vi "AR Drone + Simple nav.vi"() -> ()   [LabVIEW 2014]
doc: "Very simple example showing how to use the base VIs to control the AR Drone and receive and display video data."
uses:
  Others/Control cluster.ctl
  <vilib>/LVH/AR Drone Toolkit/Decode NavData/Typedefs/NavData Demo.ctl
  Global.vi
  <vilib>/LVH/AR Drone Toolkit/AR Drone.lvlib
panel:
  in  "milliseconds to wait":u32=5
  out "Delay (ms)":u32
  in  "Takeoff/Land":bool
  out "Video Stream 2":picture
  in  "Setup Parameters":T1={"Drone IP address"="192.168.1.1", "Home IP address"="192.168.1.2", "Flight Mode"=enum."INDOOR MODE", "Mounted Hull"=enum."INDOOR HULL", "Video Camera"=0, "Max Altitude (m)"=3.0, "Max Pitch and Roll Angle (deg)"=10.0, "Max Vertical Speed (m/s)"=0.7, "Max Yaw Speed (deg/s)"=100.0} {"Video Camera" items=["Bottom Camera"=1, "Front Camera"=0, "Front in Bottom"=3, "Bottom in Front"=2]}
  in  "stop":bool
  out "Loop error":errorcluster
  out "Loop count":i32
  out "Battery Remaining 2":dbl(slide) scale=0.0..100.0
  out "NavData Out 2":T2
  out "Control Cluster":T3 {"Yaw Speed" scale=-1.0..1.0; "Vertical Speed" scale=-1.0..1.0; "Pitch" scale=-1.0..1.0; "Roll" scale=-1.0..1.0}
  in  "Emergency Landing":bool
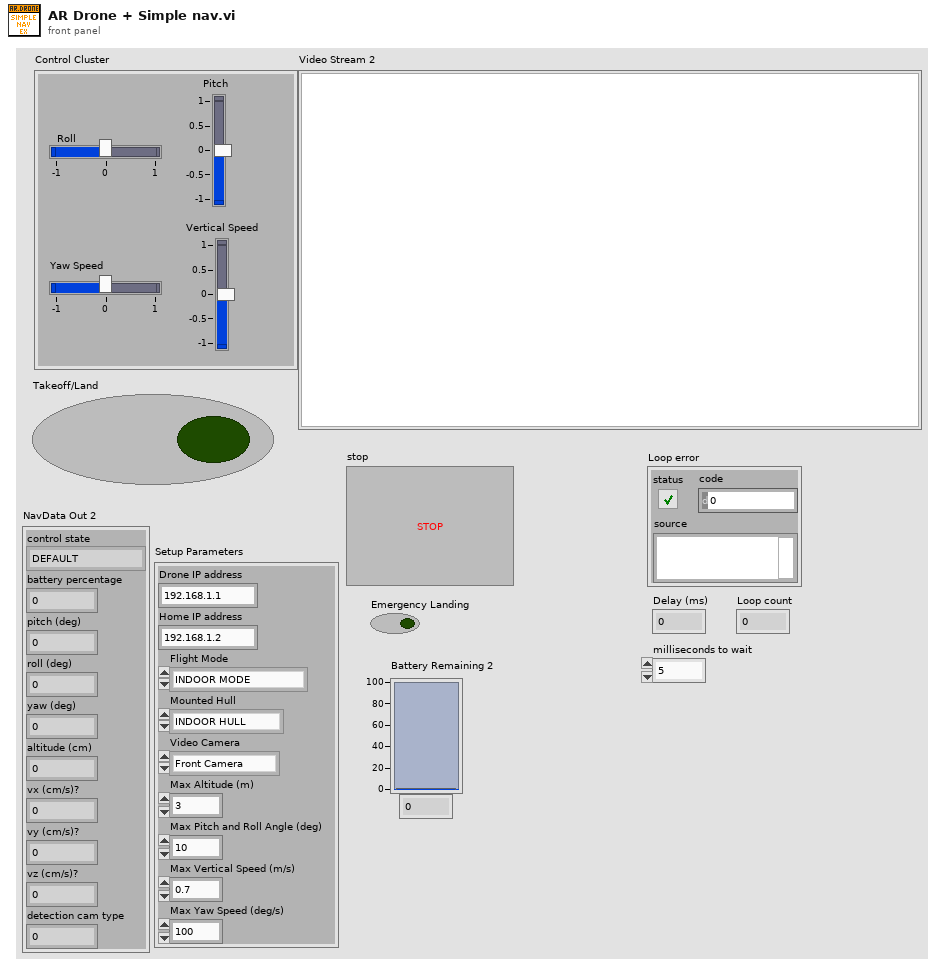
[diagram p1: front panel]
types:
  T1 = cluster{"Drone IP address":string, "Home IP address":string, "Flight Mode":enum8{"OUTDOOR MODE", "INDOOR MODE"}, "Mounted Hull":enum8{"OUTDOOR HULL", "INDOOR HULL"}, "Video Camera":u8, "Max Altitude (m)":sgl, "Max Pitch and Roll Angle (deg)":sgl, "Max Vertical Speed (m/s)":sgl, "Max Yaw Speed (deg/s)":sgl}
  T2 = typedef "AR Drone.lvlib/NavData Demo.ctl" = cluster{"control state":enum32{"DEFAULT", "INIT", "LANDING", "FLYING", "HOVERING", "TEST", "TRANS_TAKEOFF", "TRANS_GOTOFIX", "TRANS_LANDING"}, "battery percentage":u32, "pitch (deg)":sgl, "roll (deg)":sgl, "yaw (deg)":sgl, "altitude (cm)":u32, "vx (cm/s)?":sgl, "vy (cm/s)?":sgl, "vz (cm/s)?":sgl, "detection cam type":u32}
  T3 = typedef "Control cluster.ctl" = cluster{"Roll":sgl, "Pitch":sgl, "Vertical Speed":sgl, "Yaw Speed":sgl}
  T4 = typedef "AR Drone.lvlib/AR Drone Resource.ctl" = cluster{"UDP Control Connection":refnum<k16>, "UDP NavData Connection":refnum<k16>, "UDP Video Connection (Drone 1.0)":refnum<k16>, "TCP Video Connection (Drone 2.0)":refnum<k5>, "TCP Control Port Connection":refnum<k5>, "Drone IP address":string, "Drone Command Port":u16, "Drone NavData Port":u16, "Drone Vid Stream Port":u16, "Drone TCP Control Port":u16, "Home IP address":string, "Home Command Port":u16, "Home NavData Port":u16, "Home Vid Stream Port":u16, "Drone Version":i32, "Drone Index":i32, "Command Sequence":i32}
  T5 = cluster{"button 1":bool, "button 2":bool, "button 3":bool, "button 4":bool}
  T6 = cluster{"Roll":dbl, "Pitch":dbl, "Vertical Speed":dbl, "Yaw Speed":dbl}
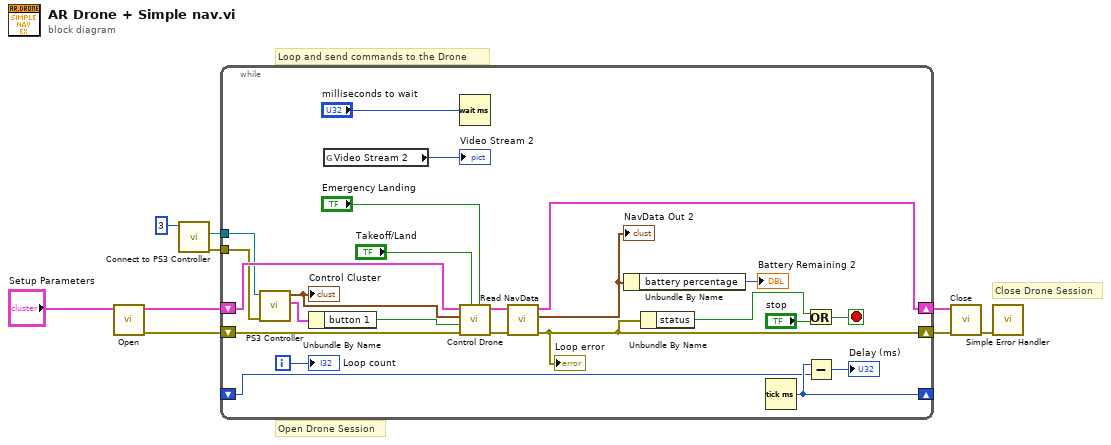
[diagram p0: block diagram]
diagram:
  # "Close Drone Session"
  # "Loop and send commands to the Drone"
  # "Open Drone Session"
  n1 = call <vilib>:"Open.vi"("Setup Parameters"="Setup Parameters") -> ("error out"=w7:errorcluster, "AR Drone Resource"=w3:T4)  [unwired: 9 in]
  n2 = call "Connect to PS3 Controller.vi"("device ID"=3) -> ("error out"=w4:errorcluster, "device ID 2"=w6:refnum<k1>)  [unwired: 7 in, 1 out]
  n3 = while {
    shift-right: [w33] -> w9
    shift-left: w3 -> [w31]
    shift-right: [w25] -> w2
    shift-left: w7 -> [w32]
    tunnel: w6 -> [w29]
    tunnel: w4 -> [w28]
    shift-right: [w12] -> _
    shift-left: _ -> [w11]
    i -> [w30]
    stop <- w26 stop-if-true
    n4 = call "PS3 Controller.vi"("error in (no error)"=w28, "device ID"=w29) -> ("Buttons control"=w23:T5, "Control cluster"=w27:T6)  [unwired: 6 in, 2 out]
    "Control Cluster" <- w27
    n5 = Unbundle By Name(w23) -> ("button 1"=w22:bool)
    n6 = global read "Global.vi" "Video Stream 2"() -> (→"Video Stream 2":picture)
    n7 = Wait (ms)(milliseconds to wait="milliseconds to wait") -> ()  [unwired: 1 out]
    n8 = call <vilib>:"Control Drone.vi"("Emergency Landing"="Emergency Landing", "Takeoff/Land"="Takeoff/Land", "error in (no error)"=w32, "Hover"=w22, "Control Cluster"=w27, "AR Drone Resource"=w31) -> ("error out"=w20:errorcluster, "AR Drone Resource Out"=w21:T4)  [unwired: 4 in]
    n9 = call <vilib>:"Read NavData.vi"("error in (no error)"=w20, "AR Drone Resource"=w21) -> ("error out"=w25:errorcluster, "NavData Out"=w13:T2, "AR Drone Resource Out"=w33:T4)  [unwired: 7 in]
    "Loop error" <- w25
    "NavData Out 2" <- w13
    n10 = Unbundle By Name(w13) -> ("battery percentage"=→"Battery Remaining 2":u32)
    n11 = Unbundle By Name(w25) -> ("status"=w16:bool)
    n12 = Tick Count (ms)() -> (millisecond timer value=w12:u32)
    n13 = Or(x=w16, y="stop") -> (x .or. y?=w26:bool)
    n14 = Subtract(x=w12, y=w11) -> (x-y=→"Delay (ms)":u32)
    "Loop count" <- w30
  }
  n15 = call <vilib>:"Close.vi"("error in (no error)"=w2, "AR Drone Resource"=w9) -> ("error out"=w8:errorcluster)  [unwired: 9 in]
  n16 = call <vilib>:"Simple Error Handler.vi"("error in (no error)"=w8) -> ()  [unwired: 4 in, 5 out]
